vi "DatabaseWrite SubVI.vi"(8 "error in (no error)":errorcluster, 9 "Image path to the user;s biometrics":string, 10 "Input second name of the new user":string, 11 "Input name of the new user":string) -> (0 "error out":errorcluster)   [LabVIEW 2024]
uses:
  <vilib>/addons/database/Connection.llb/DB Tools Open Connec (Path).vi
  <vilib>/addons/database/NI_Database_API.lvlib
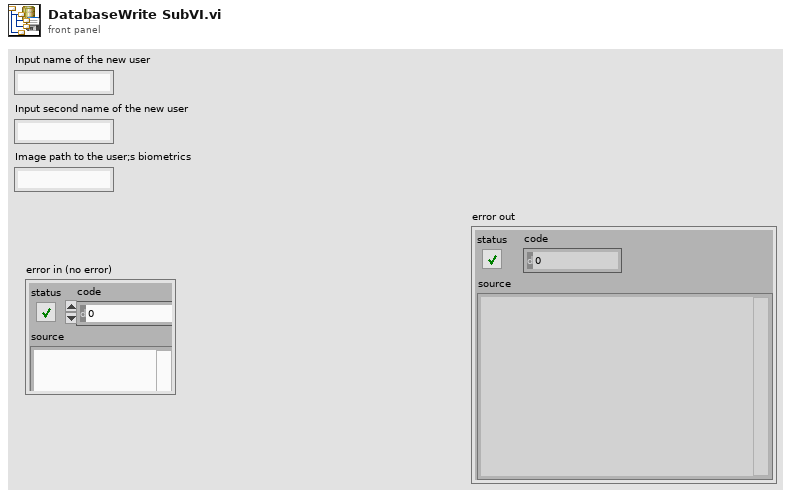
[diagram p1: front panel]
types:
  T1 = typedef "NI_Database_API.lvlib/Conn ObjectReference.ctl" = refnum<k1>
  T2 = cluster{"Input name of the new user":string, "Input second name of the new user":string, "Image path to the user;s biometrics":string, timestamp, timestamp}
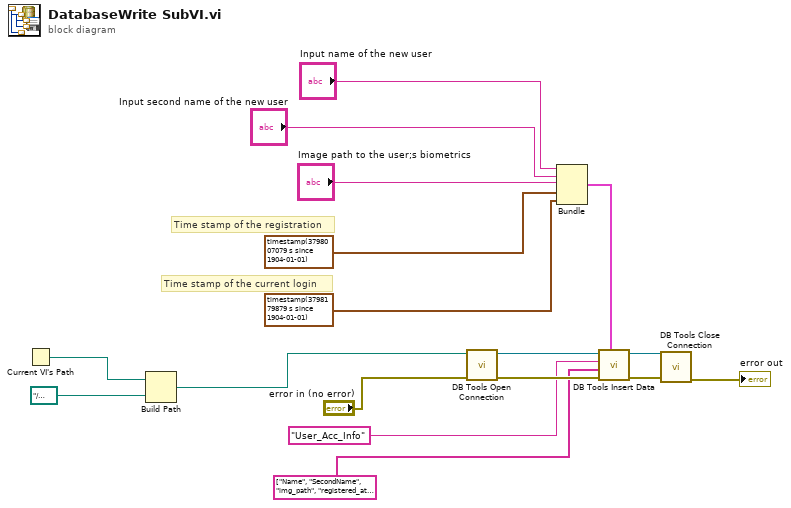
[diagram p0: block diagram]
diagram:
  # "Time stamp of the current login"
  # "Time stamp of the registration"
  n1 = Current VI's Path() -> (path=w3:path)
  n2 = Build Path(base path=w3, name or relative path=path "../conn/UserDATABASELink_upd.udl") -> (appended path=w1:path)
  n3 = call-poly <vilib>:"DB Tools Open Connection.vi"("error in (no error)"="error in (no error)", "connection information"=w1) -> ("error out"=w17:errorcluster, "connection reference"=w15:T1)  [unwired: 6 in]
  n4 = Bundle("Input name of the new user"="Input name of the new user", "Input second name of the new user"="Input second name of the new user", "Image path to the user;s biometrics"="Image path to the user;s biometrics", timestamp(3798007079 s since 1904-01-01), timestamp(3798179879 s since 1904-01-01)) -> (w11:T2)  [unwired: 1 in]
  n5 = call <vilib>:"DB Tools Insert Data.vi"("data"=w11, "error in (no error)"=w17, "columns"=string[] ["Name", "SecondName", "img_path", "registered_at", "last_logged_at"], "table"="User_Acc_Info", "connection reference"=w15) -> ("error out"=w16:errorcluster, "connection reference out"=w14:T1)  [unwired: 5 in]
  n6 = call <vilib>:"DB Tools Close Connection.vi"("error in (no error)"=w16, "connection reference"=w14) -> ("error out"=→"error out":errorcluster)  [unwired: 5 in]
